vi "Change Scope.vi"(8 "Error In":errorcluster, 9 "Data":variant, 10 "Messages In":refnum<queue>, 11 "State In":T1) -> (0 "Error Out":errorcluster, 2 "Messages Out":refnum<queue>, 3 "State Out":T1)   [LabVIEW 2018, in "Bookmark Manager.lvlib"]
uses:
  Bookmark Manager.lvlib
  Controls/State.ctl
  <vilib>/addons/analyzer/_analyzerctrls.llb/VIAnCtl Analysis App Info.ctl
  Controls/Bookmark.ctl
  Controls/VI Identifier.ctl
  Controls/Bookmarks Groups.ctl
  Controls/Message.ctl
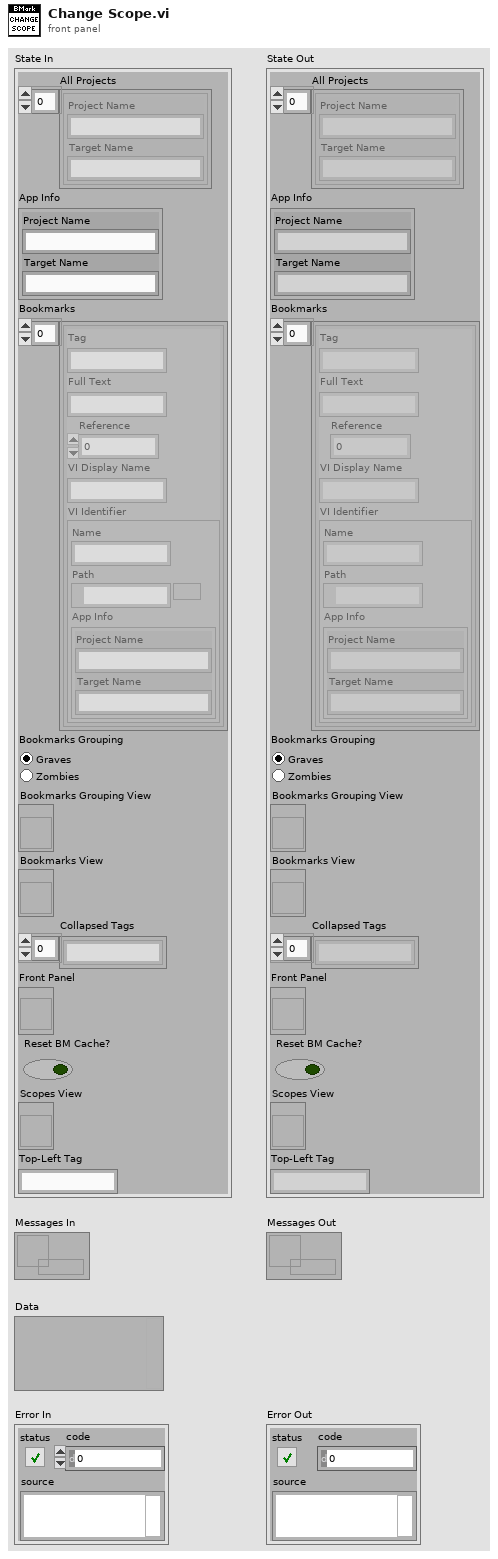
[diagram p1: front panel]
types:
  T1 = typedef "Bookmark Manager.lvlib/State.ctl" = cluster{"All Projects":T2[], "App Info":T2, "Bookmarks":T3[], "Bookmarks Grouping":T5, "Bookmarks Grouping View":refnum<vi>, "Bookmarks View":refnum<vi>, "Collapsed Tags":string[], "Front Panel":refnum<vi>, "Reset BM Cache?":bool, "Scopes View":refnum<vi>, "Top-Left Tag":string}
  T2 = typedef "VIAnCtl Analysis App Info.ctl" = cluster{"Project Name":string, "Target Name":string}
  T3 = typedef "Bookmark Manager.lvlib/Bookmark.ctl" = cluster{"Tag":string, "Full Text":string, "Reference":i32, "VI Display Name":string, "VI Identifier":T4}
  T4 = typedef "Bookmark Manager.lvlib/VI Identifier.ctl" = cluster{"Name":string, "Path":path, "App Info":T2}
  T5 = typedef "Bookmark Manager.lvlib/Bookmarks Groups.ctl" = enum32{"Graves", "Zombies"}
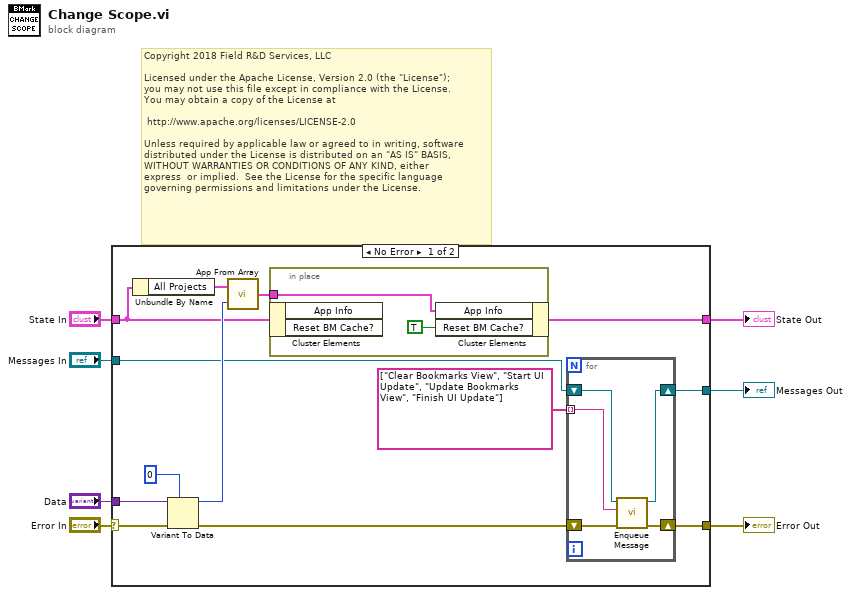
[diagram p0: block diagram]
diagram:
  # "Copyright 2018 Field R&D Services, LLC\n\nLicensed under the Apache License, Version 2.0 (the \"License\");\nyou may not use this file except in compliance with the License.\nYou may obtain a copy of the License at\n\n\thttp://www.apache.org/licenses/LICENSE-2.0\n\nUnless required by applicable law or agreed to in writing, software\ndistributed under the License is distributed on an \"AS IS\" BASIS,\nWITHOUT WARRANTIES OR CONDITIONS OF ANY KIND, either \nexpress  or implied.  See the License for the specific language \ngoverning permissions and limitations under the License."
  n1 = case shown="No Error" "Error In" {
    selector: "Error In" -> [w9 w30]
    tunnel: [w18 w30] -> w7
    tunnel: "State In" -> [w14 w29]
    tunnel: "Data" -> [w12 _]
    tunnel: [w11 w29] -> w4
    tunnel: "Messages In" -> [w10 w28]
    tunnel: [w8 w28] -> w1
    frame No Error {
      n2 = Unbundle By Name(w14) -> ("All Projects"=w15:T2[])
      n3 = Variant To Data(error in=w9, type=u16 0, Variant=w12) -> (data=w16:u16, error out=w19:errorcluster)
      n4 = call "App From Array.vi"("Projects"=w16, "All Projects"=w15) -> ("App Info"=w17:T2)
      n5 = in-place {
        in-place-border: w17 -> [w27]
        n6 = in-place-cluster #1(w14) -> ()  [unwired: 2 out]
        n7 = in-place-cluster #1("App Info"=w27, "Reset BM Cache?"=TRUE) -> (w11:T1)
      }
      n8 = for {
        shift-right: [w25] -> w18
        shift-left: w19 -> [w24]
        tunnel: string[] ["Clear Bookmarks View", "Start UI Update", "Update Bookmarks View", "Finish UI Update"] -> [w23] mode=indexing
        shift-right: [w21] -> w8
        shift-left: w10 -> [w22]
        n9 = call "Enqueue Message.vi"("Error In"=w24, "Command"=w23, "Message Queue In"=w22) -> ("Error Out"=w25:errorcluster, "Message Queue Out"=w21:refnum<queue>)  [unwired: 7 in]
      }
    }
    frame Error {
    }
  }
  "Error Out" <- w7
  "State Out" <- w4
  "Messages Out" <- w1
